vi "Kobuki Sensor Display.vi"(5 "sensors":T3 {"Kobuki Sensors"."Charger Source" items=["DISCHARGING"=0, "DOCKING_CHARGED"=2, "DOCKING_CHARGING"=6, "ADAPTER_CHARGED"=18, "ADAPTER_CHARGING"=22]; "accelerometer"."z axis (g)" format="%.3f"; "accelerometer"."y axis (g)" format="%.3f"; "accelerometer"."x axis (g)" format="%.3f"}) -> (2 "Kobuki Sensors Display":T1 {"Right Wheel (mm/s)" scale=-500.0..500.0; "Left Wheel (mm/s)" scale=-500.0..500.0})   [LabVIEW 2017]
doc: "Convert robot sensors into a graphical control for display in UI."
uses:
  Sensors.ctl
  Accelerometer.ctl
  Kobuki/KobukiSensors.ctl
  Kobuki/Kobuki Bumps and WheelDrops.ctl
  Kobuki/Kobuki Buttons.ctl
  Kobuki Sensor Display.ctl
panel:
  # "Electrical: charging, battery, OI mode"
  # "Sensors: bump, cliff, button, wheel drop"
  # "Motors:"
  # "Inertia"
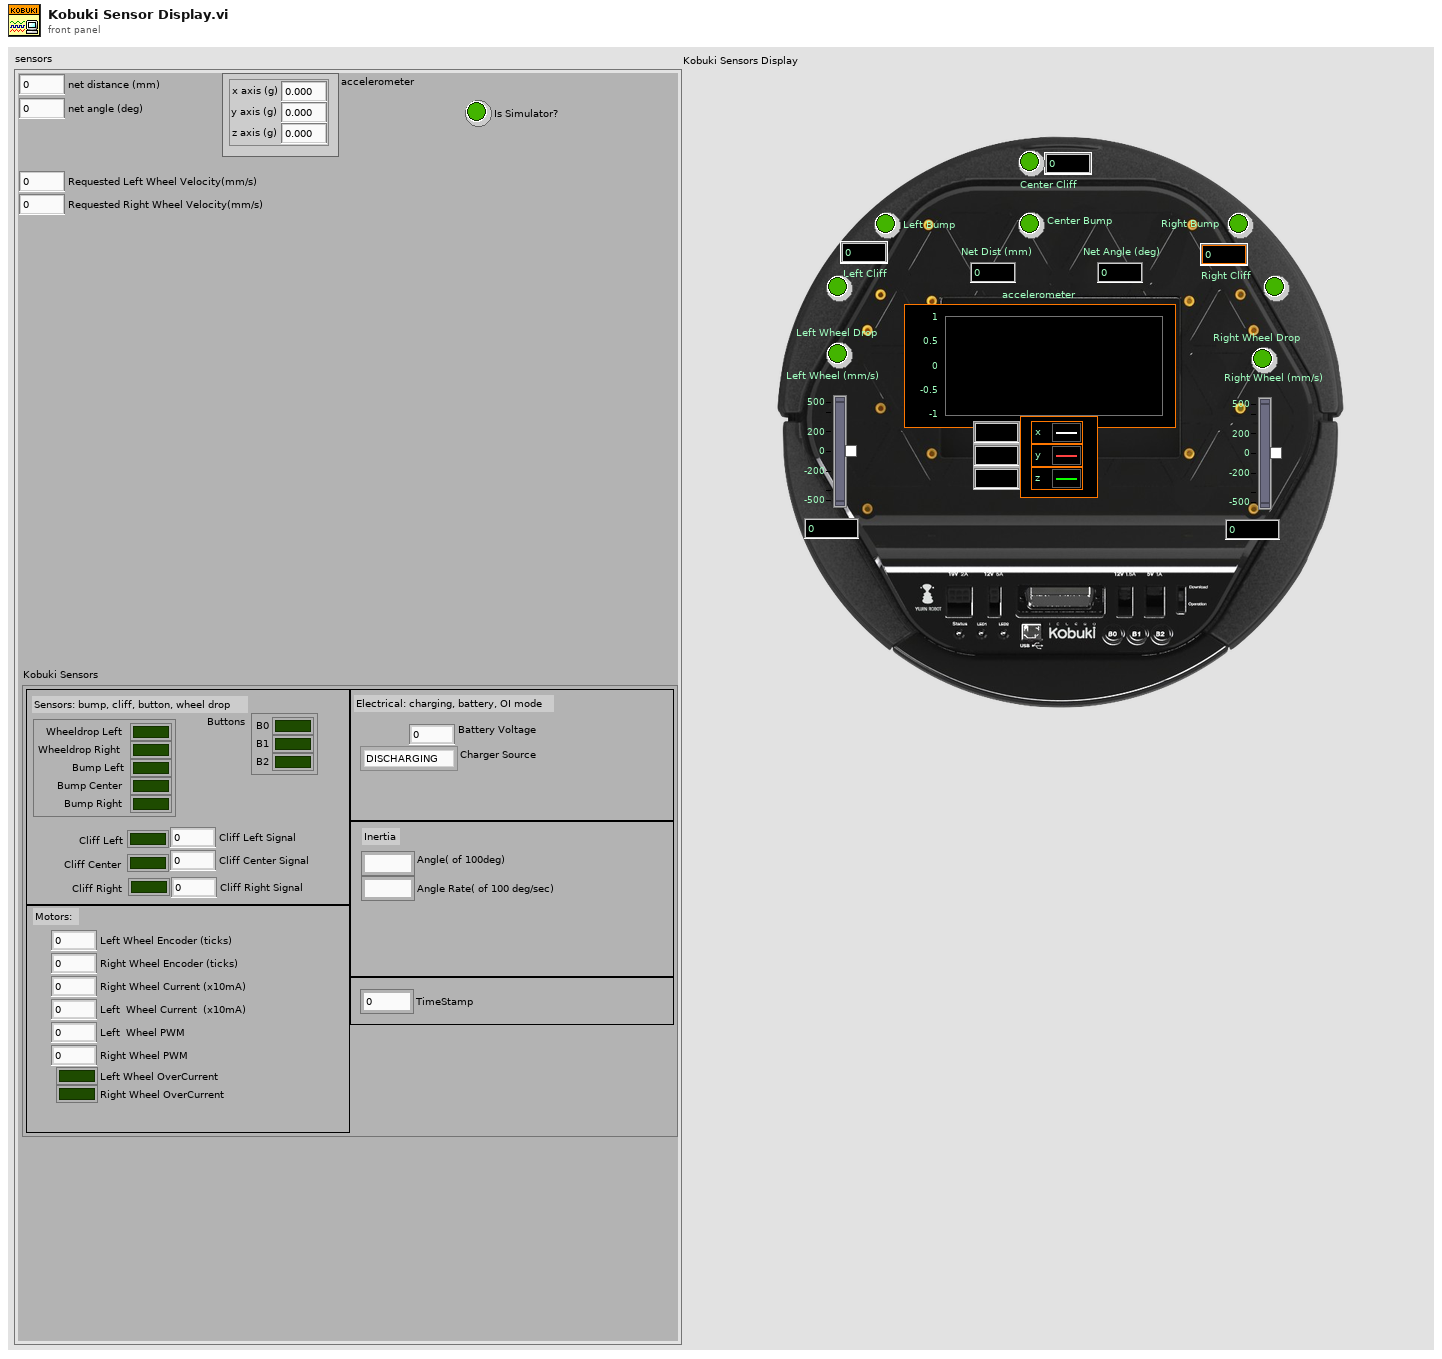
[diagram p1: front panel]
types:
  T1 = typedef "Kobuki Sensor Display.ctl" = cluster{"Center Bump":bool, "Left Wheel Drop":bool, "Right Wheel Drop":bool, "Left Bump":bool, "Right Bump":bool, "Left Cliff":bool, "Center Cliff":bool, "Right Cliff":bool, "Net Dist (mm)":i32, "Net Angle (deg)":i32, "Left Cliff":u16, "Center Cliff":u16, "Right Cliff":u16, "  Left Wheel (mm/s)":i16, "Right Wheel (mm/s)":i16, "accelerometer":T2}
  T2 = typedef "Accelerometer.ctl" = cluster{"x axis (g)":dbl, "y axis (g)":dbl, "z axis (g)":dbl}
  T3 = typedef "Sensors.ctl" = cluster{"net distance (mm)":i32, "net angle (deg)":i32, "accelerometer":T2, "Is Simulator?":bool, "Kobuki Sensors":T4, "Requested Left Wheel Velocity(mm/s)":i32, "Requested Right Wheel Velocity(mm/s)":i32}
  T4 = typedef "KobukiSensors.ctl" = cluster{"Bumps + Wheel Drops":T5, "Cliff Left":bool, "Cliff Center":bool, "Cliff Right":bool, "Cliff Left Signal":u16, "Cliff Center Signal":u16, "Cliff Right Signal":u16, "Buttons":T6, "Left Wheel Encoder (ticks)":u16, "Right Wheel Encoder (ticks) ":u16, "Left  Wheel PWM":i8, "Right Wheel PWM":i8, "Left Wheel OverCurrent":bool, "Right Wheel OverCurrent ":bool, "Right Wheel Current (x10mA)":i16, "Left  Wheel Current  (x10mA)":i16, "TimeStamp":u16, "Battery Voltage":dbl, "Angle( of 100deg)":i16, "Angle Rate( of 100 deg/sec)":i16, "Charger Source ":i8}
  T5 = typedef "Kobuki Bumps and WheelDrops.ctl" = cluster{"Wheeldrop Left":bool, "Wheeldrop Right":bool, "Bump Left":bool, "Bump Center":bool, "Bump Right":bool}
  T6 = typedef "Kobuki Buttons.ctl" = cluster{"B0":bool, "B1":bool, "B2":bool}
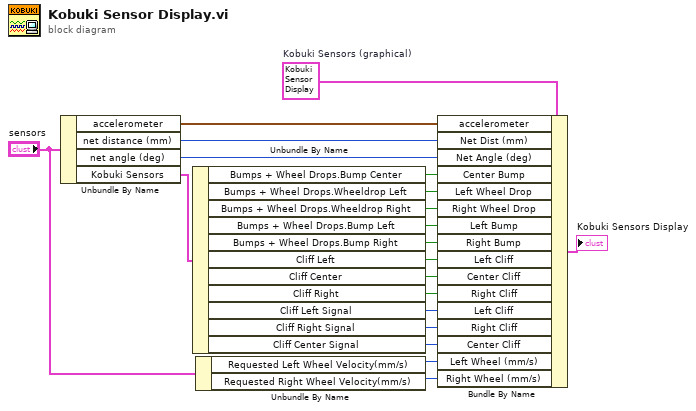
[diagram p0: block diagram]
diagram:
  w7 = T1 {"Center Bump"=FALSE, "Left Wheel Drop"=FALSE, "Right Wheel Drop"=FALSE, "Left Bump"=FALSE, "Right Bump"=FALSE, "Left Cliff"=FALSE, "Center Cliff"=FALSE, "Right Cliff"=FALSE, "Net Dist (mm)"=0, "Net Angle (deg)"=0, "Left Cliff"=0, "Center Cliff"=0, "Right Cliff"=0, "  Left Wheel (mm/s)"=0, "Right Wheel (mm/s)"=0, "accelerometer"={"x axis (g)"=0.0, "y axis (g)"=0.0, "z axis (g)"=0.0}}  # Kobuki Sensors (graphical)
  n1 = Unbundle By Name("sensors") -> ("accelerometer"=w8:T2, "net distance (mm)"=w9:i32, "net angle (deg)"=w10:i32, "Kobuki Sensors"=w11:T4)
  n2 = Unbundle By Name(w11) -> ("Bumps + Wheel Drops.Bump Center"=w20:bool, "Bumps + Wheel Drops.Wheeldrop Left"=w19:bool, "Bumps + Wheel Drops.Wheeldrop Right"=w18:bool, "Bumps + Wheel Drops.Bump Left"=w17:bool, "Bumps + Wheel Drops.Bump Right"=w16:bool, "Cliff Left"=w15:bool, "Cliff Center"=w14:bool, "Cliff Right"=w13:bool, "Cliff Left Signal"=w12:u16, "Cliff Right Signal"=w6:u16, "Cliff Center Signal"=w4:u16)
  n3 = Unbundle By Name("sensors") -> ("Requested Left Wheel Velocity(mm/s)"=w2:i32, "Requested Right Wheel Velocity(mm/s)"=w1:i32)
  n4 = Bundle By Name(cluster=w7, "accelerometer"=w8, "Net Dist (mm)"=w9, "Net Angle (deg)"=w10, "Center Bump"=w20, "Left Wheel Drop"=w19, "Right Wheel Drop"=w18, "Left Bump"=w17, "Right Bump"=w16, "Left Cliff"=w15, "Center Cliff"=w14, "Right Cliff"=w13, "Left Cliff"=w12, "Right Cliff"=w6, "Center Cliff"=w4, "Left Wheel (mm/s)"=w2, "Right Wheel (mm/s)"=w1) -> (→"Kobuki Sensors Display":T1)
